vi "SensorDataConverter.vi"(4 "RO 7":dbl, 5 "RO 0":dbl, 6 "RO 6":dbl, 7 "RO 1":dbl, 8 "RO 5":dbl, 9 "RO 4":dbl, 10 "RO 3":dbl, 11 "RO 2":dbl) -> (1 "[R] Line Present":bool, 2 "[C] Line Present":bool, 3 "[L] Line Present":bool)   [LabVIEW 2019]
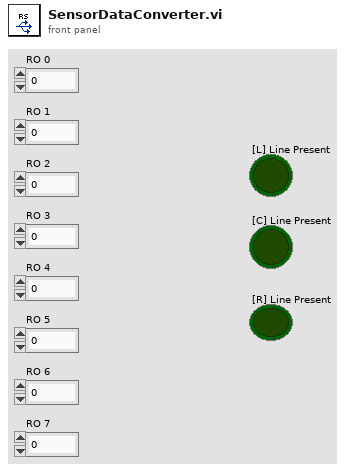
[diagram p1: front panel]
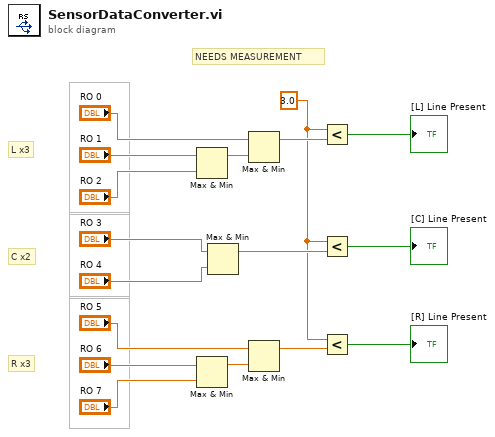
[diagram p0: block diagram]
diagram:
  w4 = 3.0
  # "NEEDS MEASUREMENT"
  # "R x3"
  # "C x2"
  # "L x3"
  n1 = Max & Min(x="RO 1", y="RO 2") -> (max(x,y)=w14:dbl)  [unwired: 1 out]
  n2 = Max & Min(x="RO 6", y="RO 7") -> (max(x,y)=w13:dbl)  [unwired: 1 out]
  n3 = Max & Min(x="RO 3", y="RO 4") -> (max(x,y)=w5:dbl)  [unwired: 1 out]
  n4 = Max & Min(x="RO 0", y=w14) -> (max(x,y)=w8:dbl)  [unwired: 1 out]
  n5 = Max & Min(x="RO 5", y=w13) -> (max(x,y)=w9:dbl)  [unwired: 1 out]
  n6 = Less?(x=w4, y=w8) -> (x < y?=→"[L] Line Present":bool)
  n7 = Less?(x=w4, y=w5) -> (x < y?=→"[C] Line Present":bool)
  n8 = Less?(x=w4, y=w9) -> (x < y?=→"[R] Line Present":bool)
